vi "CRYfinal Loudness.vi"(8 "Zwicker_X-axis":u16(ring) items=["Hz", "Bark"], 9 "SPL":dbl[](array[numeric]), 10 "Boolean":bool=TRUE, 11 "frequence":dbl[](array[numeric])) -> (0 "out Y":dbl[](array[numeric]), 1 "out X":dbl[](array[numeric]), 2 "Loud-phon":dbl, 3 "*N(sone)":dbl)   [LabVIEW 2013]
panel:
  in  "dz":dbl
  in  "iz":dbl[](array[numeric])
  in  "ig":i32
  in  "j":i32
  in  "z2":dbl
  in  "z1":dbl
  in  "N2":dbl
  in  "N1":dbl
  in  "z":dbl
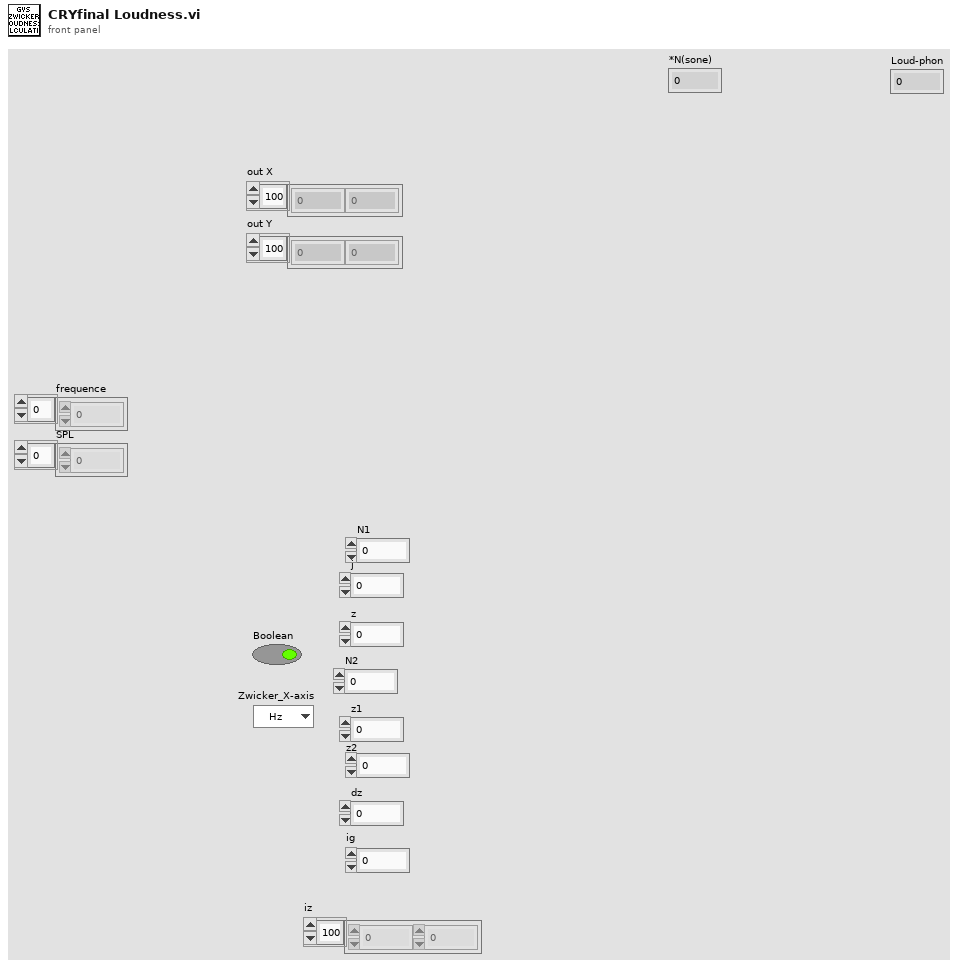
[diagram p1: front panel]
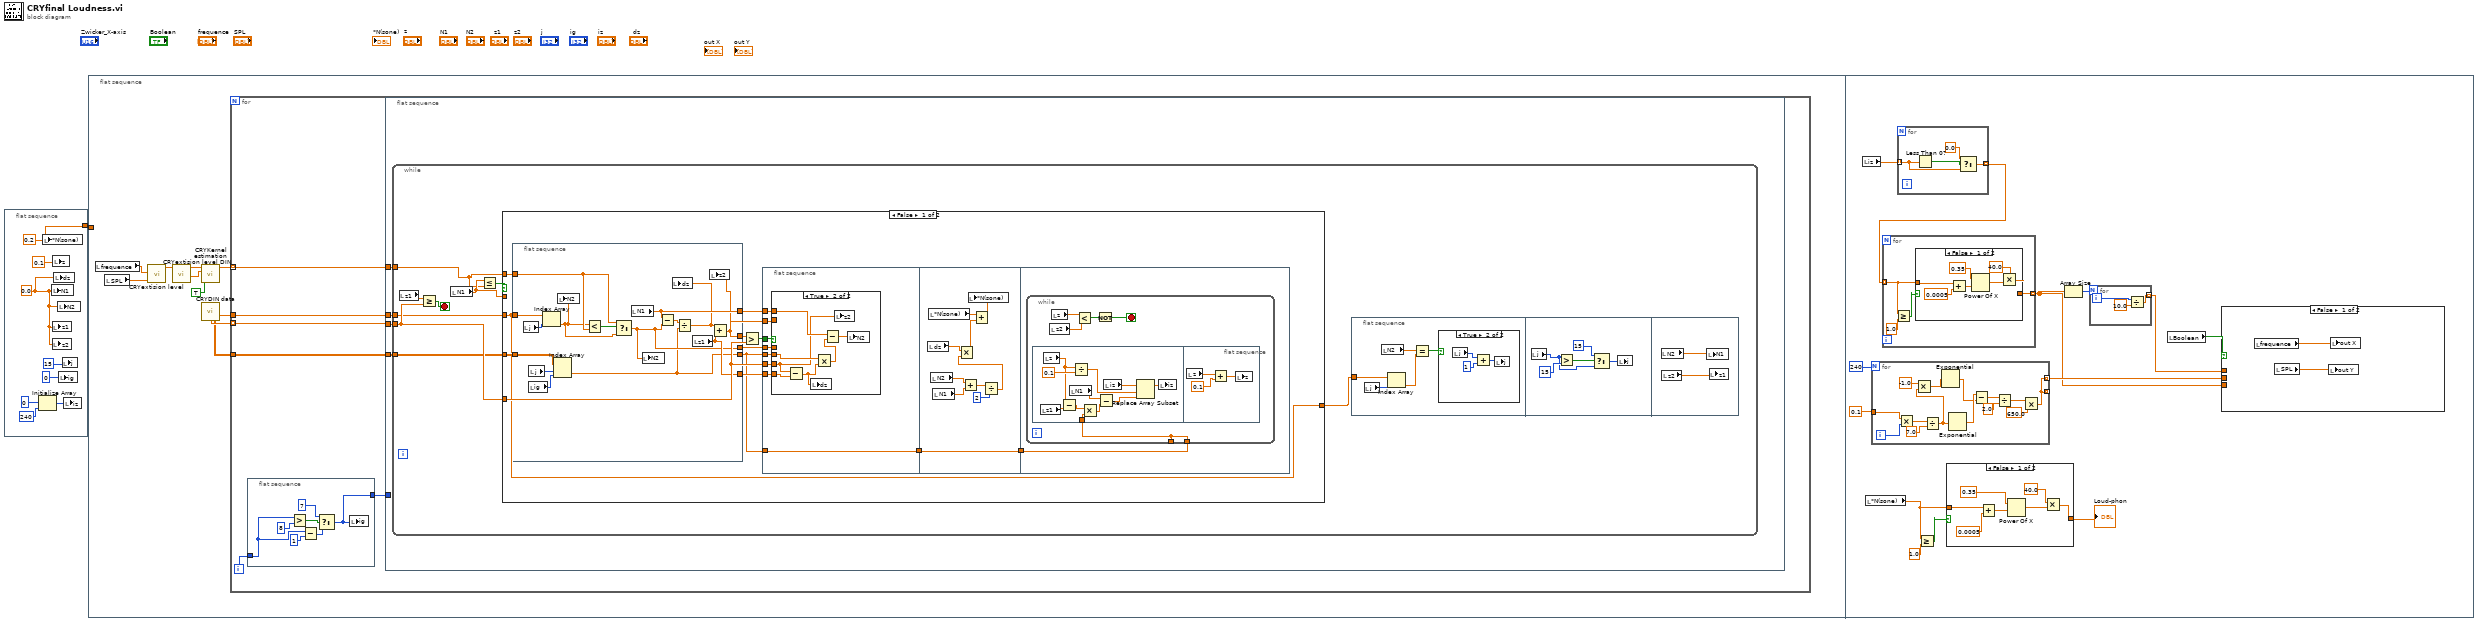
[diagram p0: block diagram]
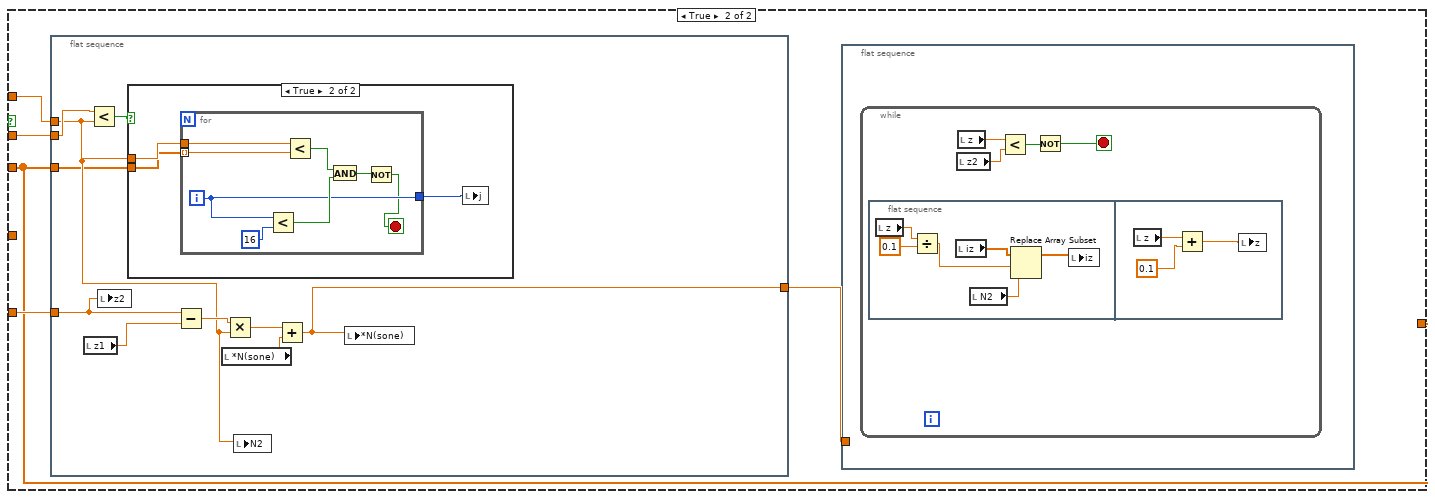
[diagram p4: hidden frame]
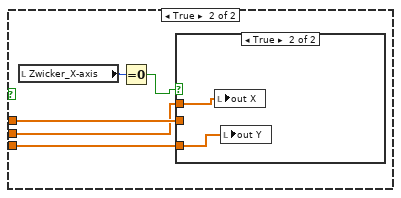
[diagram p6: hidden frame]
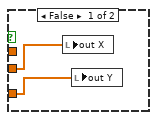
[diagram p7: hidden frame]
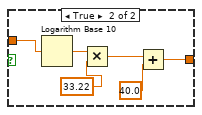
[diagram p8: hidden frame]
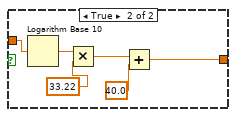
[diagram p9: hidden frame]
diagram:
  n1 = flat-sequence {
    tunnel: [w7] -> w1
    frame #0 {
      w6 = 0.0
      w7 = 0.2
      n2 = Initialize Array(0, 240) -> (w4:i32[])
      n3 = local write "*N(sone)"(w7) -> ()
      n4 = local write "N1"(w6) -> ()
      n5 = local write "z1"(w6) -> ()
      n6 = local write "z2"(w6) -> ()
      n7 = local write "z"(0.1) -> ()
      n8 = local write "dz"(w6) -> ()
      n9 = local write "N2"(w6) -> ()
      n10 = local write "ig"(0) -> ()
      n11 = local write "j"(15) -> ()
      n12 = local write "iz"(w4) -> ()
    }
  }
  n13 = flat-sequence {
    tunnel: w1 -> [_]
    frame #0 {
      n14 = local read "frequence"() -> (w11:dbl[])
      n15 = local read "SPL"() -> (w10:dbl[])
      n16 = call "CRYextision level.vi"("measured SPL"=w10, "measured frequency"=w11) -> ("extition level"=w15:dbl[])  [unwired: 6 in]
      n17 = call "CRYextision level DIN.vi"("extition level"=w15) -> ("LE"=w14:dbl[], "Ti"=w13:dbl[])  [unwired: 8 in]
      n18 = call "CRYDIN data.vi"() -> ("Upper Slopes1"=w17:dbl[][], "Slope Threshold1"=w18:dbl[], "UpperLimit of CriticalBands1"=w19:dbl[])  [unwired: 8 in, 5 out]
      n19 = call "CRYKernel estimation.vi"("free or diffuse"=TRUE, "Ti-11"=w13, "LE"=w14) -> ("Kern"=w12:dbl[])  [unwired: 8 in]
      n20 = for {
        tunnel: w19 -> [w25] mode=indexing
        tunnel: w12 -> [w24] mode=indexing
        tunnel: w18 -> [w21]
        tunnel: w17 -> [w23]
        i -> [w22]
        n21 = flat-sequence {
          tunnel: w22 -> [w167]
          tunnel: [w165] -> w20
          frame #0 {
            n22 = Greater?(x=w167, y=8) -> (0:w170:bool)
            n23 = Subtract(x=w167, y=1) -> (x-y=w166:i32)
            n24 = Select(t=7, s=w170, f=w166) -> (s? t:f=w165:i32)
            n25 = local write "ig"(w165) -> ()
          }
        }
        n26 = flat-sequence {
          tunnel: w25 -> [w29]
          tunnel: w24 -> [w28]
          tunnel: w23 -> [w27]
          tunnel: w21 -> [w26]
          tunnel: w20 -> [_]
          frame #0 {
            n27 = while {
              tunnel: w29 -> [w36]
              tunnel: w28 -> [w32]
              tunnel: w26 -> [w31]
              tunnel: w27 -> [w34]
              stop <- w38 stop-if-true
              n28 = local read "z1"() -> (w35:dbl)
              n29 = Greater Or Equal?(x=w35, y=w36) -> (x >= y?=w38:bool)
              n30 = local read "N1"() -> (w33:dbl)
              n31 = Less Or Equal?(x=w33, y=w32) -> (x <= y?=w37:bool)
              n32 = case shown="False" w37 {
                tunnel: w32 -> [w65 w128]
                tunnel: w33 -> [_ w130]
                tunnel: w31 -> [w57 w126]
                tunnel: w36 -> [w63 w129]
                tunnel: w34 -> [w64 _]
                tunnel: [w57 w126] -> w30
                frame False {
                  n33 = flat-sequence {
                    tunnel: w65 -> [w78]
                    tunnel: w64 -> [w76]
                    tunnel: [w73] -> w62
                    tunnel: [w72] -> w61
                    tunnel: [w70] -> w59
                    tunnel: [w69] -> w58
                    tunnel: w57 -> [w67]
                    tunnel: [w66] -> w54
                    frame #0 {
                      n34 = local read "j"() -> (w80:i32)
                      n35 = local read "ig"() -> (w74:i32)
                      n36 = local read "j"() -> (w75:i32)
                      n37 = Index Array(array=w67, index=w80) -> (element=w71:dbl)
                      n38 = Index Array(array=w76, index (row)=w75, index (col)=w74) -> (element=w66:dbl)
                      n39 = local write "N2"(w71) -> ()
                      n40 = Less?(x=w71, y=w78) -> (x < y?=w79:bool)
                      n41 = Select(t=w78, s=w79, f=w71) -> (s? t:f=w70:dbl)
                      n42 = local read "N1"() -> (w73:dbl)
                      n43 = local write "N2"(w70) -> ()
                      n44 = Subtract(x=w73, y=w70) -> (x-y=w77:dbl)
                      n45 = Divide(x=w77, y=w66) -> (x/y=w68:dbl)
                      n46 = local write "dz"(w68) -> ()
                      n47 = local read "z1"() -> (w72:dbl)
                      n48 = Add(x=w68, y=w72) -> (x+y=w69:dbl)
                      n49 = local write "z2"(w69) -> ()
                    }
                  }
                  n50 = Greater?(x=w58, y=w63) -> (0:w60:bool)
                  n51 = flat-sequence {
                    tunnel: w63 -> [w88]
                    tunnel: w62 -> [w87]
                    tunnel: w61 -> [w86]
                    tunnel: w54 -> [w85]
                    tunnel: w59 -> [w84]
                    tunnel: w58 -> [w83]
                    tunnel: w60 -> [w82]
                    tunnel: [w81] -> w55
                    tunnel: w54 -> [w81]
                    tunnel: [w96] -> w56
                    tunnel: w55 -> [w96]
                    tunnel: w56 -> [w106]
                    frame #0 {
                      n52 = case shown="True" w82 {
                        tunnel: w88 -> [_ w89]
                        tunnel: w87 -> [_ w94]
                        tunnel: w86 -> [_ w91]
                        tunnel: w85 -> [_ w95]
                        tunnel: w84 -> [_ _]
                        tunnel: w83 -> [_ _]
                        frame False {
                        }
                        frame True {
                          n53 = Subtract(x=w89, y=w91) -> (x-y=w90:dbl)
                          n54 = local write "dz"(w90) -> ()
                          n55 = Multiply(x=w95, y=w90) -> (x*y=w93:dbl)
                          n56 = Subtract(x=w94, y=w93) -> (x-y=w92:dbl)
                          n57 = local write "z2"(w89) -> ()
                          n58 = local write "N2"(w92) -> ()
                        }
                      }
                    }
                    frame #1 {
                      n59 = local read "dz"() -> (w98:dbl)
                      n60 = local read "*N(sone)"() -> (w105:dbl)
                      n61 = local read "N2"() -> (w104:dbl)
                      n62 = local read "N1"() -> (w103:dbl)
                      n63 = Add(x=w104, y=w103) -> (x+y=w102:dbl)
                      n64 = Divide(x=w102, y=2) -> (x/y=w100:dbl)
                      n65 = Multiply(x=w98, y=w100) -> (x*y=w99:dbl)
                      n66 = Add(x=w105, y=w99) -> (x+y=w97:dbl)
                      n67 = local write "*N(sone)"(w97) -> ()
                    }
                    frame #2 {
                      n68 = while {
                        tunnel: [w107] -> _
                        tunnel: w106 -> [w107]
                        stop <- w108 stop-if-true
                        n69 = flat-sequence {
                          tunnel: w107 -> [w116]
                          frame #0 {
                            n70 = local read "z1"() -> (w119:dbl)
                            n71 = local read "z"() -> (w114:dbl)
                            n72 = Subtract(x=w114, y=w119) -> (x-y=w117:dbl)
                            n73 = local read "N1"() -> (w118:dbl)
                            n74 = Divide(x=w114, y=0.1) -> (x/y=w120:dbl)
                            n75 = Multiply(x=w117, y=w116) -> (x*y=w115:dbl)
                            n76 = Subtract(x=w118, y=w115) -> (x-y=w113:dbl)
                            n77 = local read "iz"() -> (w122:dbl[])
                            n78 = Replace Array Subset(array=w122, new element=w113, index=w120) -> (w112:dbl[])
                            n79 = local write "iz"(w112) -> ()
                          }
                          frame #1 {
                            n80 = local read "z"() -> (w125:dbl)
                            n81 = Add(x=w125, y=0.1) -> (x+y=w123:dbl)
                            n82 = local write "z"(w123) -> ()
                          }
                        }
                        n83 = local read "z2"() -> (w111:dbl)
                        n84 = local read "z"() -> (w110:dbl)
                        n85 = Less?(x=w110, y=w111) -> (x < y?=w109:bool)
                        n86 = Not(x=w109) -> (.not. x?=w108:bool)
                      }
                    }
                  }
                }
                frame True {
                  n87 = flat-sequence {
                    tunnel: w130 -> [w149]
                    tunnel: w129 -> [w148]
                    tunnel: w128 -> [w147]
                    tunnel: w126 -> [w144]
                    tunnel: [w145] -> w127
                    frame #0 {
                      n88 = local read "z1"() -> (w146:dbl)
                      n89 = Less?(x=w149, y=w147) -> (x < y?=w153:bool)
                      n90 = local write "z2"(w148) -> ()
                      n91 = case shown="True" w153 {
                        tunnel: w147 -> [_ w156]
                        tunnel: w144 -> [_ w155]
                        frame False {
                        }
                        frame True {
                          n92 = for {
                            tunnel: w156 -> [w159]
                            tunnel: w155 -> [w158] mode=indexing
                            tunnel: [w161] -> w154
                            i -> [w161]
                            stop <- w160 stop-if-true
                            n93 = Less?(x=w161, y=16) -> (x < y?=w163:bool)
                            n94 = Less?(x=w159, y=w158) -> (x < y?=w157:bool)
                            n95 = And(x=w157, y=w163) -> (x .and. y?=w162:bool)
                            n96 = Not(x=w162) -> (.not. x?=w160:bool)
                          }
                          n97 = local write "j"(w154) -> ()
                        }
                      }
                      n98 = Subtract(x=w148, y=w146) -> (x-y=w152:dbl)
                      n99 = local read "*N(sone)"() -> (w150:dbl)
                      n100 = Multiply(x=w152, y=w147) -> (x*y=w151:dbl)
                      n101 = local write "N2"(w147) -> ()
                      n102 = Add(x=w151, y=w150) -> (x+y=w145:dbl)
                      n103 = local write "*N(sone)"(w145) -> ()
                    }
                  }
                  n104 = flat-sequence {
                    tunnel: w127 -> [_]
                    frame #0 {
                      n105 = while {
                        stop <- w131 stop-if-true
                        n106 = flat-sequence {
                          frame #0 {
                            n107 = local read "z"() -> (w138:dbl)
                            n108 = Divide(x=w138, y=0.1) -> (x/y=w136:dbl)
                            n109 = local read "iz"() -> (w140:dbl[])
                            n110 = local read "N2"() -> (w137:dbl)
                            n111 = Replace Array Subset(array=w140, new element=w137, index=w136) -> (w135:dbl[])
                            n112 = local write "iz"(w135) -> ()
                          }
                          frame #1 {
                            n113 = local read "z"() -> (w142:dbl)
                            n114 = Add(x=w142, y=0.1) -> (x+y=w141:dbl)
                            n115 = local write "z"(w141) -> ()
                          }
                        }
                        n116 = local read "z2"() -> (w134:dbl)
                        n117 = local read "z"() -> (w133:dbl)
                        n118 = Less?(x=w133, y=w134) -> (x < y?=w132:bool)
                        n119 = Not(x=w132) -> (.not. x?=w131:bool)
                      }
                    }
                  }
                }
              }
              n120 = flat-sequence {
                tunnel: w30 -> [w39]
                frame #0 {
                  n121 = local read "j"() -> (w42:i32)
                  n122 = local read "N2"() -> (w43:dbl)
                  n123 = Index Array(array=w39, index=w42) -> (element=w41:dbl)
                  n124 = Equal?(x=w43, y=w41) -> (x = y?=w40:bool)
                  n125 = case shown="True" w40 {
                    frame False {
                    }
                    frame True {
                      n126 = local read "j"() -> (w46:i32)
                      n127 = Add(x=w46, y=1) -> (x+y=w44:i32)
                      n128 = local write "j"(w44) -> ()
                    }
                  }
                }
                frame #1 {
                  n129 = local read "j"() -> (w47:i32)
                  n130 = Greater?(x=w47, y=15) -> (0:w50:bool)
                  n131 = Select(t=15, s=w50, f=w47) -> (s? t:f=w49:i32)
                  n132 = local write "j"(w49) -> ()
                }
                frame #2 {
                  n133 = local read "N2"() -> (w52:dbl)
                  n134 = local read "z2"() -> (w53:dbl)
                  n135 = local write "N1"(w52) -> ()
                  n136 = local write "z1"(w53) -> ()
                }
              }
            }
          }
        }
      }
    }
    frame #1 {
      n137 = local read "iz"() -> (w173:dbl[])
      n138 = local read "*N(sone)"() -> (w181:dbl)
      n139 = for {
        N: 240 -> [_]
        tunnel: 0.1 -> [w212]
        tunnel: [w200] -> _ mode=indexing
        tunnel: [w200] -> w175 mode=indexing
        i -> [w213]
        n140 = Multiply(x=w212, y=w213) -> (x*y=w201:dbl)
        n141 = Divide(x=w201, y=7.0) -> (x/y=w209:dbl)
        n142 = Multiply(x=-1.0, y=w209) -> (x*y=w208:dbl)
        n143 = Exponential(1:w208) -> (0:w206:dbl)
        n144 = Exponential(1:w209) -> (0:w207:dbl)
        n145 = Subtract(x=w207, y=w206) -> (x-y=w205:dbl)
        n146 = Divide(x=w205, y=2.0) -> (x/y=w203:dbl)
        n147 = Multiply(x=w203, y=650.0) -> (x*y=w200:dbl)
      }
      n148 = for {
        tunnel: w173 -> [w186] mode=indexing
        tunnel: [w185] -> w172 mode=indexing
        n149 = Less Than 0?(x=w186) -> (x < 0?=w188:bool)
        n150 = Select(t=0.0, s=w188, f=w186) -> (s? t:f=w185:dbl)
      }
      n151 = for {
        tunnel: w172 -> [w218] mode=indexing
        tunnel: [w217] -> w174 mode=indexing
        n152 = Greater Or Equal?(x=w218, y=1.0) -> (x >= y?=w219:bool)
        n153 = case shown="False" w219 {
          tunnel: w218 -> [w227 w233]
          tunnel: [w221 w228] -> w217
          frame False {
            n154 = Add(x=w227, y=0.0005) -> (x+y=w225:dbl)
            n155 = Power Of X(1:w225, 2:0.35) -> (0:w223:dbl)
            n156 = Multiply(x=40.0, y=w223) -> (x*y=w221:dbl)
          }
          frame True {
            n157 = Logarithm Base 10(1:w233) -> (0:w232:dbl)
            n158 = Multiply(x=w232, y=33.22) -> (x*y=w230:dbl)
            n159 = Add(x=w230, y=40.0) -> (x+y=w228:dbl)
          }
        }
      }
      n160 = Greater Or Equal?(x=w181, y=1.0) -> (x >= y?=w184:bool)
      n161 = case shown="False" w184 {
        tunnel: w181 -> [w240 w246]
        tunnel: [w234 w241] -> w182
        frame False {
          n162 = Add(x=w240, y=0.0005) -> (x+y=w238:dbl)
          n163 = Power Of X(1:w238, 2:0.35) -> (0:w236:dbl)
          n164 = Multiply(x=40.0, y=w236) -> (x*y=w234:dbl)
        }
        frame True {
          n165 = Logarithm Base 10(1:w246) -> (0:w245:dbl)
          n166 = Multiply(x=w245, y=33.22) -> (x*y=w243:dbl)
          n167 = Add(x=w243, y=40.0) -> (x+y=w241:dbl)
        }
      }
      "Loud-phon" <- w182
      n168 = Array Size(array=w174) -> (size(s)=w180:i32)
      n169 = for {
        N: w180 -> [_]
        tunnel: [w214] -> w176 mode=indexing
        i -> [w216]
        n170 = Divide(x=w216, y=10.0) -> (x/y=w214:dbl)
      }
      n171 = local read "Boolean"() -> (w177:bool)
      n172 = case shown="False" w177 {
        tunnel: w176 -> [_ w193]
        tunnel: w174 -> [_ w192]
        tunnel: w175 -> [_ w191]
        frame False {
          n173 = local read "frequence"() -> (w190:dbl[])
          n174 = local read "SPL"() -> (w189:dbl[])
          n175 = local write "out Y"(w189) -> ()
          n176 = local write "out X"(w190) -> ()
        }
        frame True {
          n177 = local read "Zwicker_X-axis"() -> (w195:u16)
          n178 = Equal To 0?(x=w195) -> (x = 0?=w194:bool)
          n179 = case shown="True" w194 {
            tunnel: w192 -> [w197 w199]
            tunnel: w193 -> [w196 _]
            tunnel: w191 -> [_ w198]
            frame False {
              n180 = local write "out X"(w196) -> ()
              n181 = local write "out Y"(w197) -> ()
            }
            frame True {
              n182 = local write "out X"(w198) -> ()
              n183 = local write "out Y"(w199) -> ()
            }
          }
        }
      }
    }
  }
